vi "findDynamicIPToChange.vi"() -> ()   [LabVIEW 2016]
uses:
  <vilib>/Rock Robotics/Network Tables/NT Write String.vi
panel:
  out "IP":string
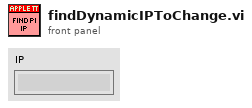
[diagram p1: front panel]
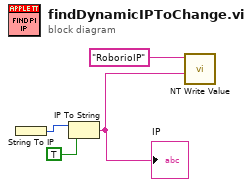
[diagram p0: block diagram]
diagram:
  n1 = String To IP() -> (0:w4:u32)  [unwired: 1 in]
  n2 = IP To String(1:TRUE ("dot notation? (F)"), 2:w4) -> (0:w2:string)
  "IP" <- w2
  n3 = call-poly <vilib>:"NT Write Value.vi"("String"=w2, "Name"="RoborioIP") -> ()  [unwired: 9 in, 1 out]
